vi "Save Type-Specific Macro Parameters.vi"(7 "Section":string, 8 "error in (no error)":errorcluster, 10 "Macro Step":T1={"Type"=enum."Mouse Move", "X"=0, "Y"=0, "Delay"=0, "Key"=65, "Repeat"=0, "RClick?"=FALSE, "App/Window Name"="", "Notes"="", "Assertion Type"=enum."Control Position", "Assertion Parameters"=variant}, 11 "refnum":T4) -> (0 "error out":errorcluster, 3 "refnum out":T4)   [LabVIEW 2020, in "MacroAssert.lvlib"]
doc: "Saves the list of steps to the macro config file defined by <B>refnum</B>."
uses:
  MacroAssert.lvlib
  <vilib>/Utility/config.llb/NI_LVConfig.lvlib
  <vilib>/Utility/config.llb/Write Key (Boolean).vi
  <vilib>/Utility/config.llb/Write Key (U32).vi
  <vilib>/Utility/config.llb/Write Key (String).vi
  <vilib>/Utility/config.llb/Write Key (I32).vi
  <vilib>/Utility/config.llb/Config Data RefNum.ctl
  CTLs/Step Type V3.ctl
  CTLs/Step V3.ctl
  CTLs/Assertion Type.ctl
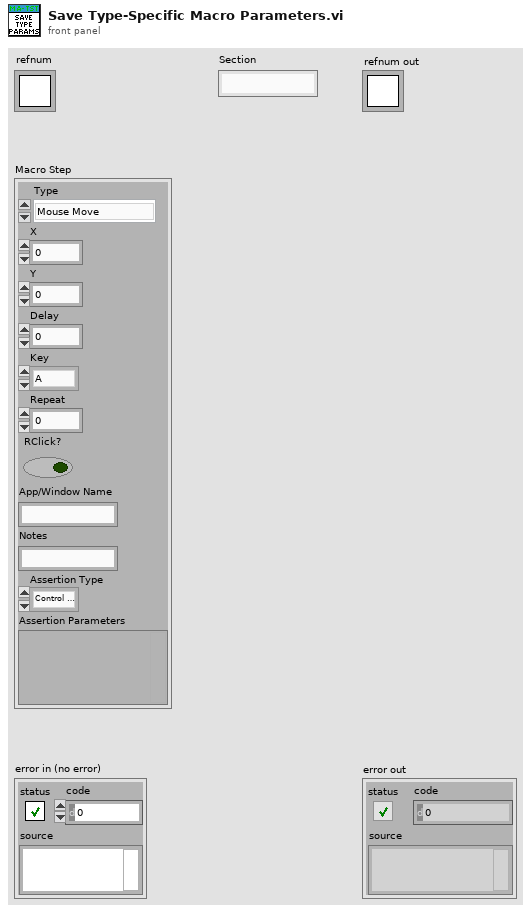
[diagram p1: front panel]
types:
  T1 = typedef "MacroAssert.lvlib/Step V3.ctl" = cluster{"Type":T2, "X":i32, "Y":i32, "Delay":i32, "Key":u8, "Repeat":i32, "RClick?":bool, "App/Window Name":string, "Notes":string, "Assertion Type":T3, "Assertion Parameters":variant}
  T2 = typedef "MacroAssert.lvlib/Step Type V3.ctl" = enum16{"Mouse Move", "Mouse Click", "Key Press", "Wait", "Mouse Down", "Mouse Up", "Key Down", "Key Up", "Test Assertion", "Run Application", "Maximize Window", "Restore Window", "Minimize Window", "Close Window", "Bring Window to Front", "Send Window to Back"}
  T3 = typedef "MacroAssert.lvlib/Assertion Type.ctl" = enum16{"Control Position", "Control Visible", "Control Disabled"}
  T4 = typedef "NI_LVConfig.lvlib/Config Data RefNum.ctl" = refnum<k1>
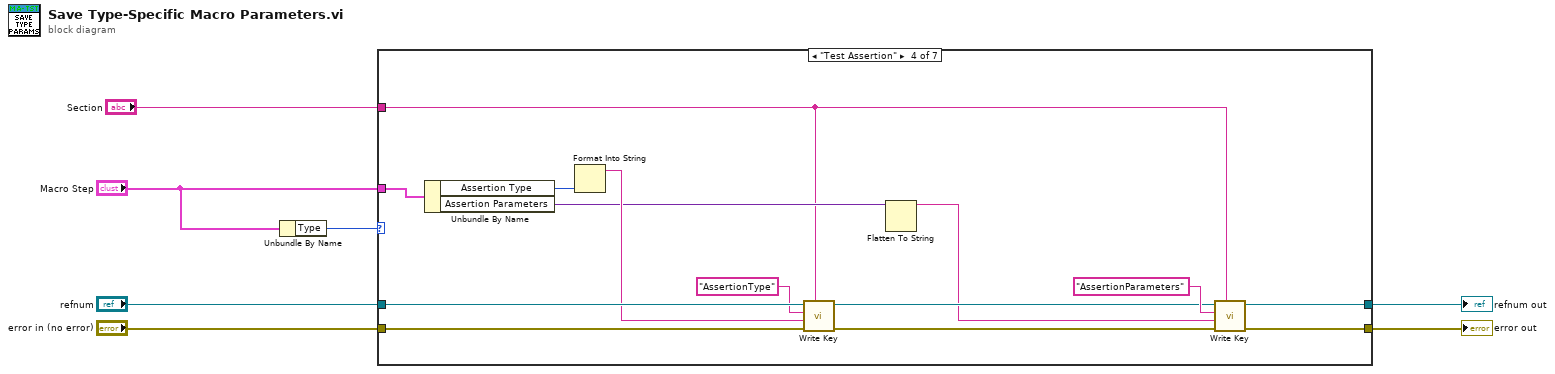
[diagram p0: block diagram]
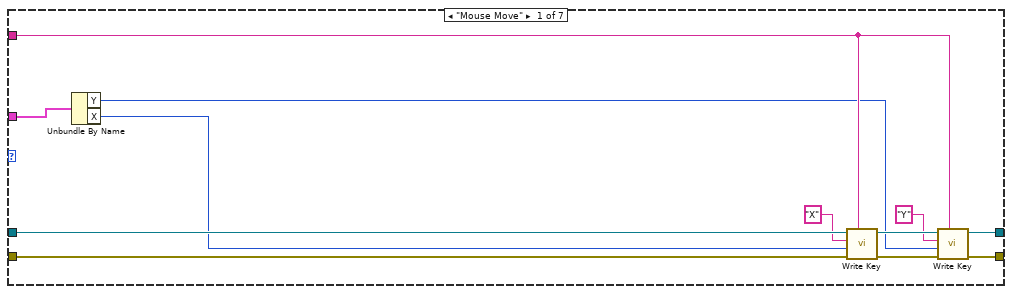
[diagram p2: hidden frame]
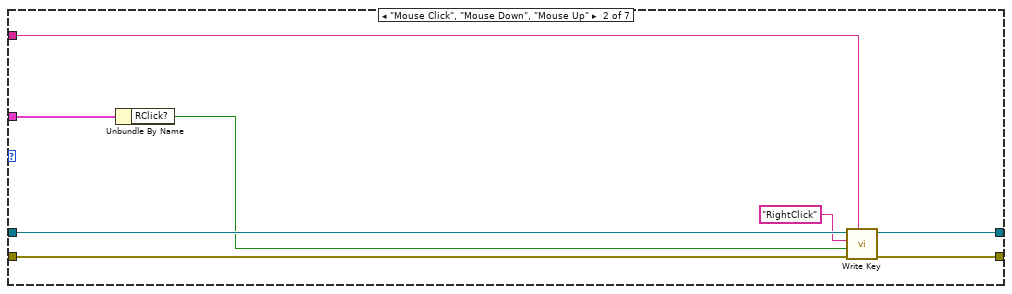
[diagram p3: hidden frame]
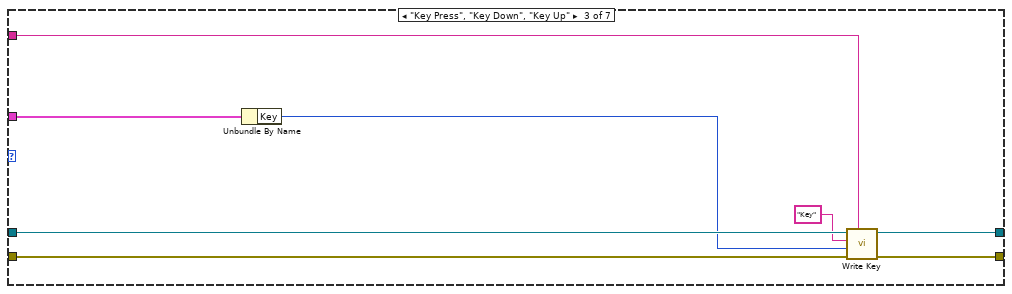
[diagram p4: hidden frame]
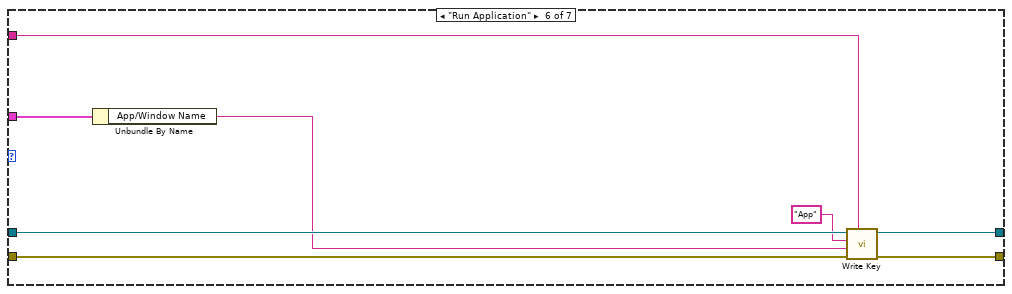
[diagram p6: hidden frame]
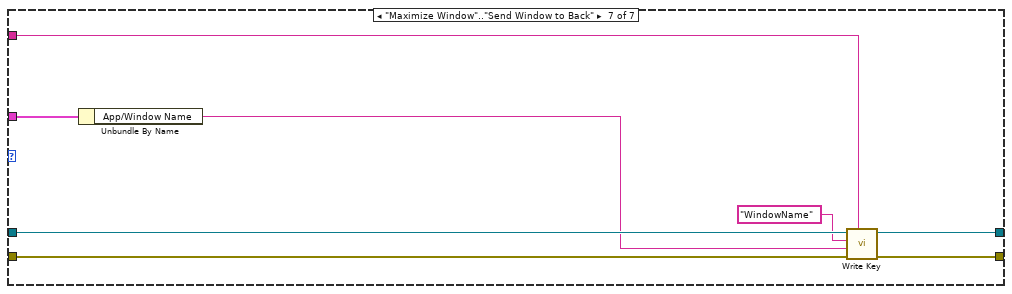
[diagram p7: hidden frame]
diagram:
  n1 = Unbundle By Name("Macro Step") -> ("Type"=w2:T2)
  n2 = case shown="\"Test Assertion\"" w2 {
    tunnel: "error in (no error)" -> [w18 w27 w35 w49 w50 w59 w67]
    tunnel: "refnum" -> [w17 w26 w34 w48 w51 w58 w66]
    tunnel: "Section" -> [w13 w24 w32 w36 _ w56 w64]
    tunnel: [w12 w22 w30 w39 w50 w54 w62] -> w5
    tunnel: [w11 w23 w31 w40 w51 w55 w63] -> w4
    tunnel: "Macro Step" -> [w10 w21 w29 w46 _ w53 w61]
    frame "Mouse Move" {
      n3 = Unbundle By Name(w10) -> ("Y"=w8:i32, "X"=w9:i32)
      n4 = call-poly <vilib>:"Write Key.vi"("section"=w13, "error in (no error)"=w18, "value"=w9, "key"="X", "refnum"=w17) -> ("error out"=w14:errorcluster, "refnum out"=w19:T4)  [unwired: 4 in, 1 out]
      n5 = call-poly <vilib>:"Write Key.vi"("section"=w13, "error in (no error)"=w14, "value"=w8, "key"="Y", "refnum"=w19) -> ("error out"=w12:errorcluster, "refnum out"=w11:T4)  [unwired: 4 in, 1 out]
    }
    frame "Mouse Click", "Mouse Down", "Mouse Up" {
      n6 = Unbundle By Name(w21) -> ("RClick?"=w20:bool)
      n7 = call-poly <vilib>:"Write Key.vi"("section"=w24, "error in (no error)"=w27, "value"=w20, "key"="RightClick", "refnum"=w26) -> ("error out"=w22:errorcluster, "refnum out"=w23:T4)  [unwired: 4 in, 1 out]
    }
    frame "Key Press", "Key Down", "Key Up" {
      n8 = Unbundle By Name(w29) -> ("Key"=w28:u8)
      n9 = call-poly <vilib>:"Write Key.vi"("section"=w32, "error in (no error)"=w35, "value"=w28, "key"="Key", "refnum"=w34) -> ("error out"=w30:errorcluster, "refnum out"=w31:T4)  [unwired: 4 in, 1 out]
    }
    frame "Test Assertion" {
      n10 = Unbundle By Name(w46) -> ("Assertion Type"=w45:T3, "Assertion Parameters"=w38:variant)
      n11 = Format Into String(w45) -> (resulting string=w44:string)  [unwired: 3 in, 1 out]
      n12 = call-poly <vilib>:"Write Key.vi"("section"=w36, "error in (no error)"=w49, "value"=w44, "key"="AssertionType", "refnum"=w48) -> ("error out"=w41:errorcluster, "refnum out"=w42:T4)  [unwired: 4 in, 1 out]
      n13 = Flatten To String(anything=w38) -> (data string=w37:string)  [unwired: 3 in, 2 out]
      n14 = call-poly <vilib>:"Write Key.vi"("section"=w36, "error in (no error)"=w41, "value"=w37, "key"="AssertionParameters", "refnum"=w42) -> ("error out"=w39:errorcluster, "refnum out"=w40:T4)  [unwired: 4 in, 1 out]
    }
    frame "Wait" {
    }
    frame "Run Application" {
      n15 = Unbundle By Name(w53) -> ("App/Window Name"=w52:string)
      n16 = call-poly <vilib>:"Write Key.vi"("section"=w56, "error in (no error)"=w59, "value"=w52, "key"="App", "refnum"=w58) -> ("error out"=w54:errorcluster, "refnum out"=w55:T4)  [unwired: 4 in, 1 out]
    }
    frame "Maximize Window".."Send Window to Back" {
      n17 = Unbundle By Name(w61) -> ("App/Window Name"=w60:string)
      n18 = call-poly <vilib>:"Write Key.vi"("section"=w64, "error in (no error)"=w67, "value"=w60, "key"="WindowName", "refnum"=w66) -> ("error out"=w62:errorcluster, "refnum out"=w63:T4)  [unwired: 4 in, 1 out]
    }
  }
  "error out" <- w5
  "refnum out" <- w4
